vi "Periodic Tasks.vi"(8 "error in":errorcluster) -> ()   [LabVIEW 2014]
doc: "This VI runs in parallel to other tasks. It can contain as many user-defined periodic loops as you need. These can carry out PID or other sorts of timed response."
uses:
  <vilib>/Rock Robotics/WPI/Solenoid/WPI_SolenoidValue.ctl
  <vilib>/Rock Robotics/WPI/Relay/WPI_RelayValue.ctl
  <vilib>/Rock Robotics/WPI/DriverStation/WPI_DriverStationRobotMode2.ctl
  TORC Code/DriveSwitch.ctl
  Robot Global Data.vi
  TORC Code/GlobalVariable.vi
  <vilib>/Rock Robotics/WPI/Solenoid/WPI_SolenoidSetEnum.vi
  <vilib>/Rock Robotics/WPI/Solenoid/Deprecated/WPI_SolenoidGetBool.vi
  <vilib>/Rock Robotics/WPI/RobotDrive/WPI_RobotDriveGetSetRefNum.vi
  <vilib>/Rock Robotics/WPI/Joystick/WPI_JoystickGetSetRefNum.vi
  <vilib>/Rock Robotics/WPI/Compressor/WPI_CompressorGetSetRefNum.vi
  <vilib>/Rock Robotics/Network Tables/SD Write Numeric Array.vi
  <vilib>/Rock Robotics/Network Tables/SD Write Boolean Array.vi
  Moose Code/Auto_Conf.vi
panel:
  out "Right Distance":dbl
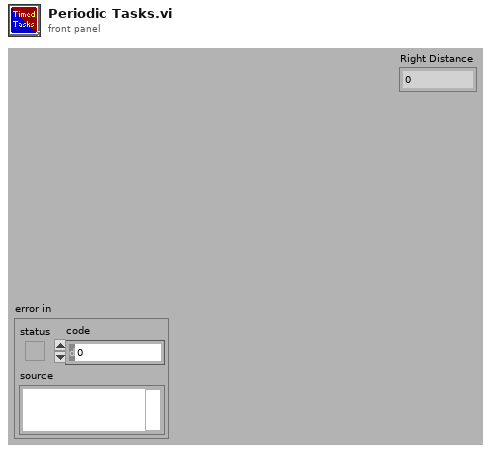
[diagram p1: front panel]
types:
  T1 = enum16{"Unready", "Ready", "Clear", "Fire", "Reload", "Arm In"}
  T2 = typedef "WPI_JoystickDevRef.ctl" = cluster{"Device":T3}
  T3 = typedef "WPI_JoystickDeviceEnum.ctl" = enum16{"USB 0", "USB 1", "USB 2", "USB 3", "USB 4", "USB 5"}
  T4 = typedef "WPI_SolenoidDevRef.ctl" = cluster{"DevStatus":errorcluster, "Pneumatics Control Module":u8, "Forward Solenoid Channel":T5, "Reverse Solenoid Channel":T5}
  T5 = typedef "WPI_SolenoidChannel.ctl" = enum8{"Solenoid 0", "Solenoid 1", "Solenoid 2", "Solenoid 3", "Solenoid 4", "Solenoid 5", "Solenoid 6", "Solenoid 7", "Invalid"}
  T6 = typedef "WPI_AnalogChannelDevRef.ctl" = cluster{"DevStatus":errorcluster, "Controller":T7, "Analog Channel":T8}
  T7 = typedef "FPGA_TypedefAnalogModule.ctl" = enum16{"Controller 1"}
  T8 = typedef "FPGA_AIChannel.ctl" = enum8{"AI 0", "AI 1", "AI 2", "AI 3", "AI MXP 0", "AI MXP 1", "AI MXP 2", "AI MXP 3", "Invalid"}
  T9 = typedef "WPI_DigitalInputDevRef.ctl" = cluster{"DevStatus":errorcluster, "DIO Channel":T10, "Controller":T11}
  T10 = typedef "FPGA_DIOChannel.ctl" = enum8{"DIO 0", "DIO 1", "DIO 2", "DIO 3", "DIO 4", "DIO 5", "DIO 6", "DIO 7", "DIO 8", "DIO 9", "DIO MXP 0", "DIO MXP 1", "DIO MXP 2", "DIO MXP 3", "DIO MXP 4", "DIO MXP 5", "DIO MXP 6", "DIO MXP 7", "DIO MXP 8", "DIO MXP 9", "DIO MXP 10", "DIO MXP 11", "DIO MXP 12", "DIO MXP 13", "DIO MXP 14", "DIO MXP 15", "Invalid"}
  T11 = typedef "FPGA_TypedefDigitalModule.ctl" = enum16{"Controller 1"}
  T12 = typedef "WPI_RobotDriveDevRef.ctl" = cluster{"DevStatus":errorcluster, "Motors[]":T13[], "Square Inputs":bool, "Max Output":dbl}
  T13 = typedef "WPI_MotorControlDeviceRef.ctl" = cluster{"DeviceStatus":errorcluster, "Type":T14, "PWM":cluster{"Controller":T11, "PWM Channel":T15, "DeadBand":T16}, "CAN":cluster{"Device Number":u8, "Control Mode":T17, "Semaphore":T18, "Max Vout":dbl, "TalonSRX Control Mode":T19}, "Invert":bool, "TransformRef":T20, "InvTransformRef":T20}
  T14 = typedef "WPI_MotorControlType.ctl" = enum16{"PWM", "CAN", "CANTalonSRX"}
  T15 = typedef "FPGA_DIOPWMChannel.ctl" = enum8{"PWM 0", "PWM 1", "PWM 2", "PWM 3", "PWM 4", "PWM 5", "PWM 6", "PWM 7", "PWM 8", "PWM 9", "PWM MXP 0", "PWM MXP 1", "PWM MXP 2", "PWM MXP 3", "PWM MXP 4", "PWM MXP 5", "PWM MXP 6", "PWM MXP 7", "PWM MXP 8", "PWM MXP 9", "Invalid"}
  T16 = typedef "WPI_PWMDeadband.ctl" = cluster{"Name":string, "maxPositivePwm":i32, "minPositivePwm":i32, "centerPwm":i32, "maxNegativePwm":i32, "minNegativePwm":i32, "angularRange":u16}
  T17 = typedef "WPI_CANJaguar_ControlMode.ctl" = enum8{"Percent VBus", "Current", "Speed", "Position", "Voltage"}
  T18 = typedef "Semaphore RefNum" = refnum<k1>
  T19 = typedef "WPI_CANTalonSRX_APIControlMode.ctl" = enum8{"Percent VBus", "Speed", "Position", "Slave", "Unchanged / Invalid"}
  T20 = typedef "WPI_PWMTransform_ConPane.ctl" = refnum<vi>
  T21 = typedef "WPI_GyroDevRef.ctl" = cluster{"DevStatus":errorcluster, "Analog Module":T7, "Analog Channel":T8, "Offset":dbl, "Gain (VoltsPerDegree/Second)":dbl}
  T22 = typedef "WPI_RelayDevRef.ctl" = cluster{"DevStatus":errorcluster, "Relay Channel":T23, "Controller":T11, "Relay Direction":T24}
  T23 = typedef "FPGA_DIORelayChannel.ctl" = enum8{"Relay 0", "Relay 1", "Relay 2", "Relay 3", "Invalid"}
  T24 = typedef "WPI_RelayDirection.ctl" = enum16{"Both directions", "Forward only", "Reverse only"}
  T25 = typedef "WPI_EncoderDevRef.ctl" = cluster{"DevStatus":errorcluster, "EncoderIndex":T26, "CounterIndex":T27, "DistancePerCount":dbl, "Decoding Type":T28}
  T26 = typedef "FPGA_EncoderIdx.ctl" = enum8{"Enc 0", "Enc 1", "Enc 2", "Enc 3", "Enc 4", "Enc 5", "Enc 6", "Enc 7", "Invalid"}
  T27 = typedef "FPGA_CounterCtrSystemIndex.ctl" = enum8{"Ctr 0", "Ctr 1", "Ctr 2", "Ctr 3", "Ctr 4", "Ctr 5", "Ctr 6", "Ctr 7", "Invalid"}
  T28 = typedef "WPI_EncoderType.ctl" = enum16{"1x", "2x", "4x"}
  T29 = typedef "WPI_CompressorDevRef.ctl" = cluster{"DevStatus":errorcluster, "Pneumatics Control Module":u8}
  T30 = typedef "WPI_DriverStationRobotMode2.ctl" = enum16{"Autonomous Disabled", "Autonomous Enabled", "Teleop Disabled", "Teleop Enabled", "Disconnected", "Finish", "Test Disabled", "Test Enabled", "Emergency Stopped"}
  T31 = typedef "WPI_RelayValue.ctl" = enum16{"Off", "On", "Forward", "Reverse"}
  T32 = typedef "WPI_SolenoidValue.ctl" = enum16{"Off", "On", "Forward", "Reverse"}
  T33 = cluster{"Buttons[0]":bool, "Buttons[1]":bool, "Buttons[2]":bool, "Buttons[3]":bool, "Buttons[4]":bool, "Buttons[5]":bool, "Buttons[6]":bool, "Buttons[7]":bool, "Buttons[8]":bool}
  T34 = typedef "DriveSwitch.ctl" = enum16{"High", "Low", "Auto"}
  T35 = typedef "Shift Enum.ctl" = enum16{"High", "Low"}
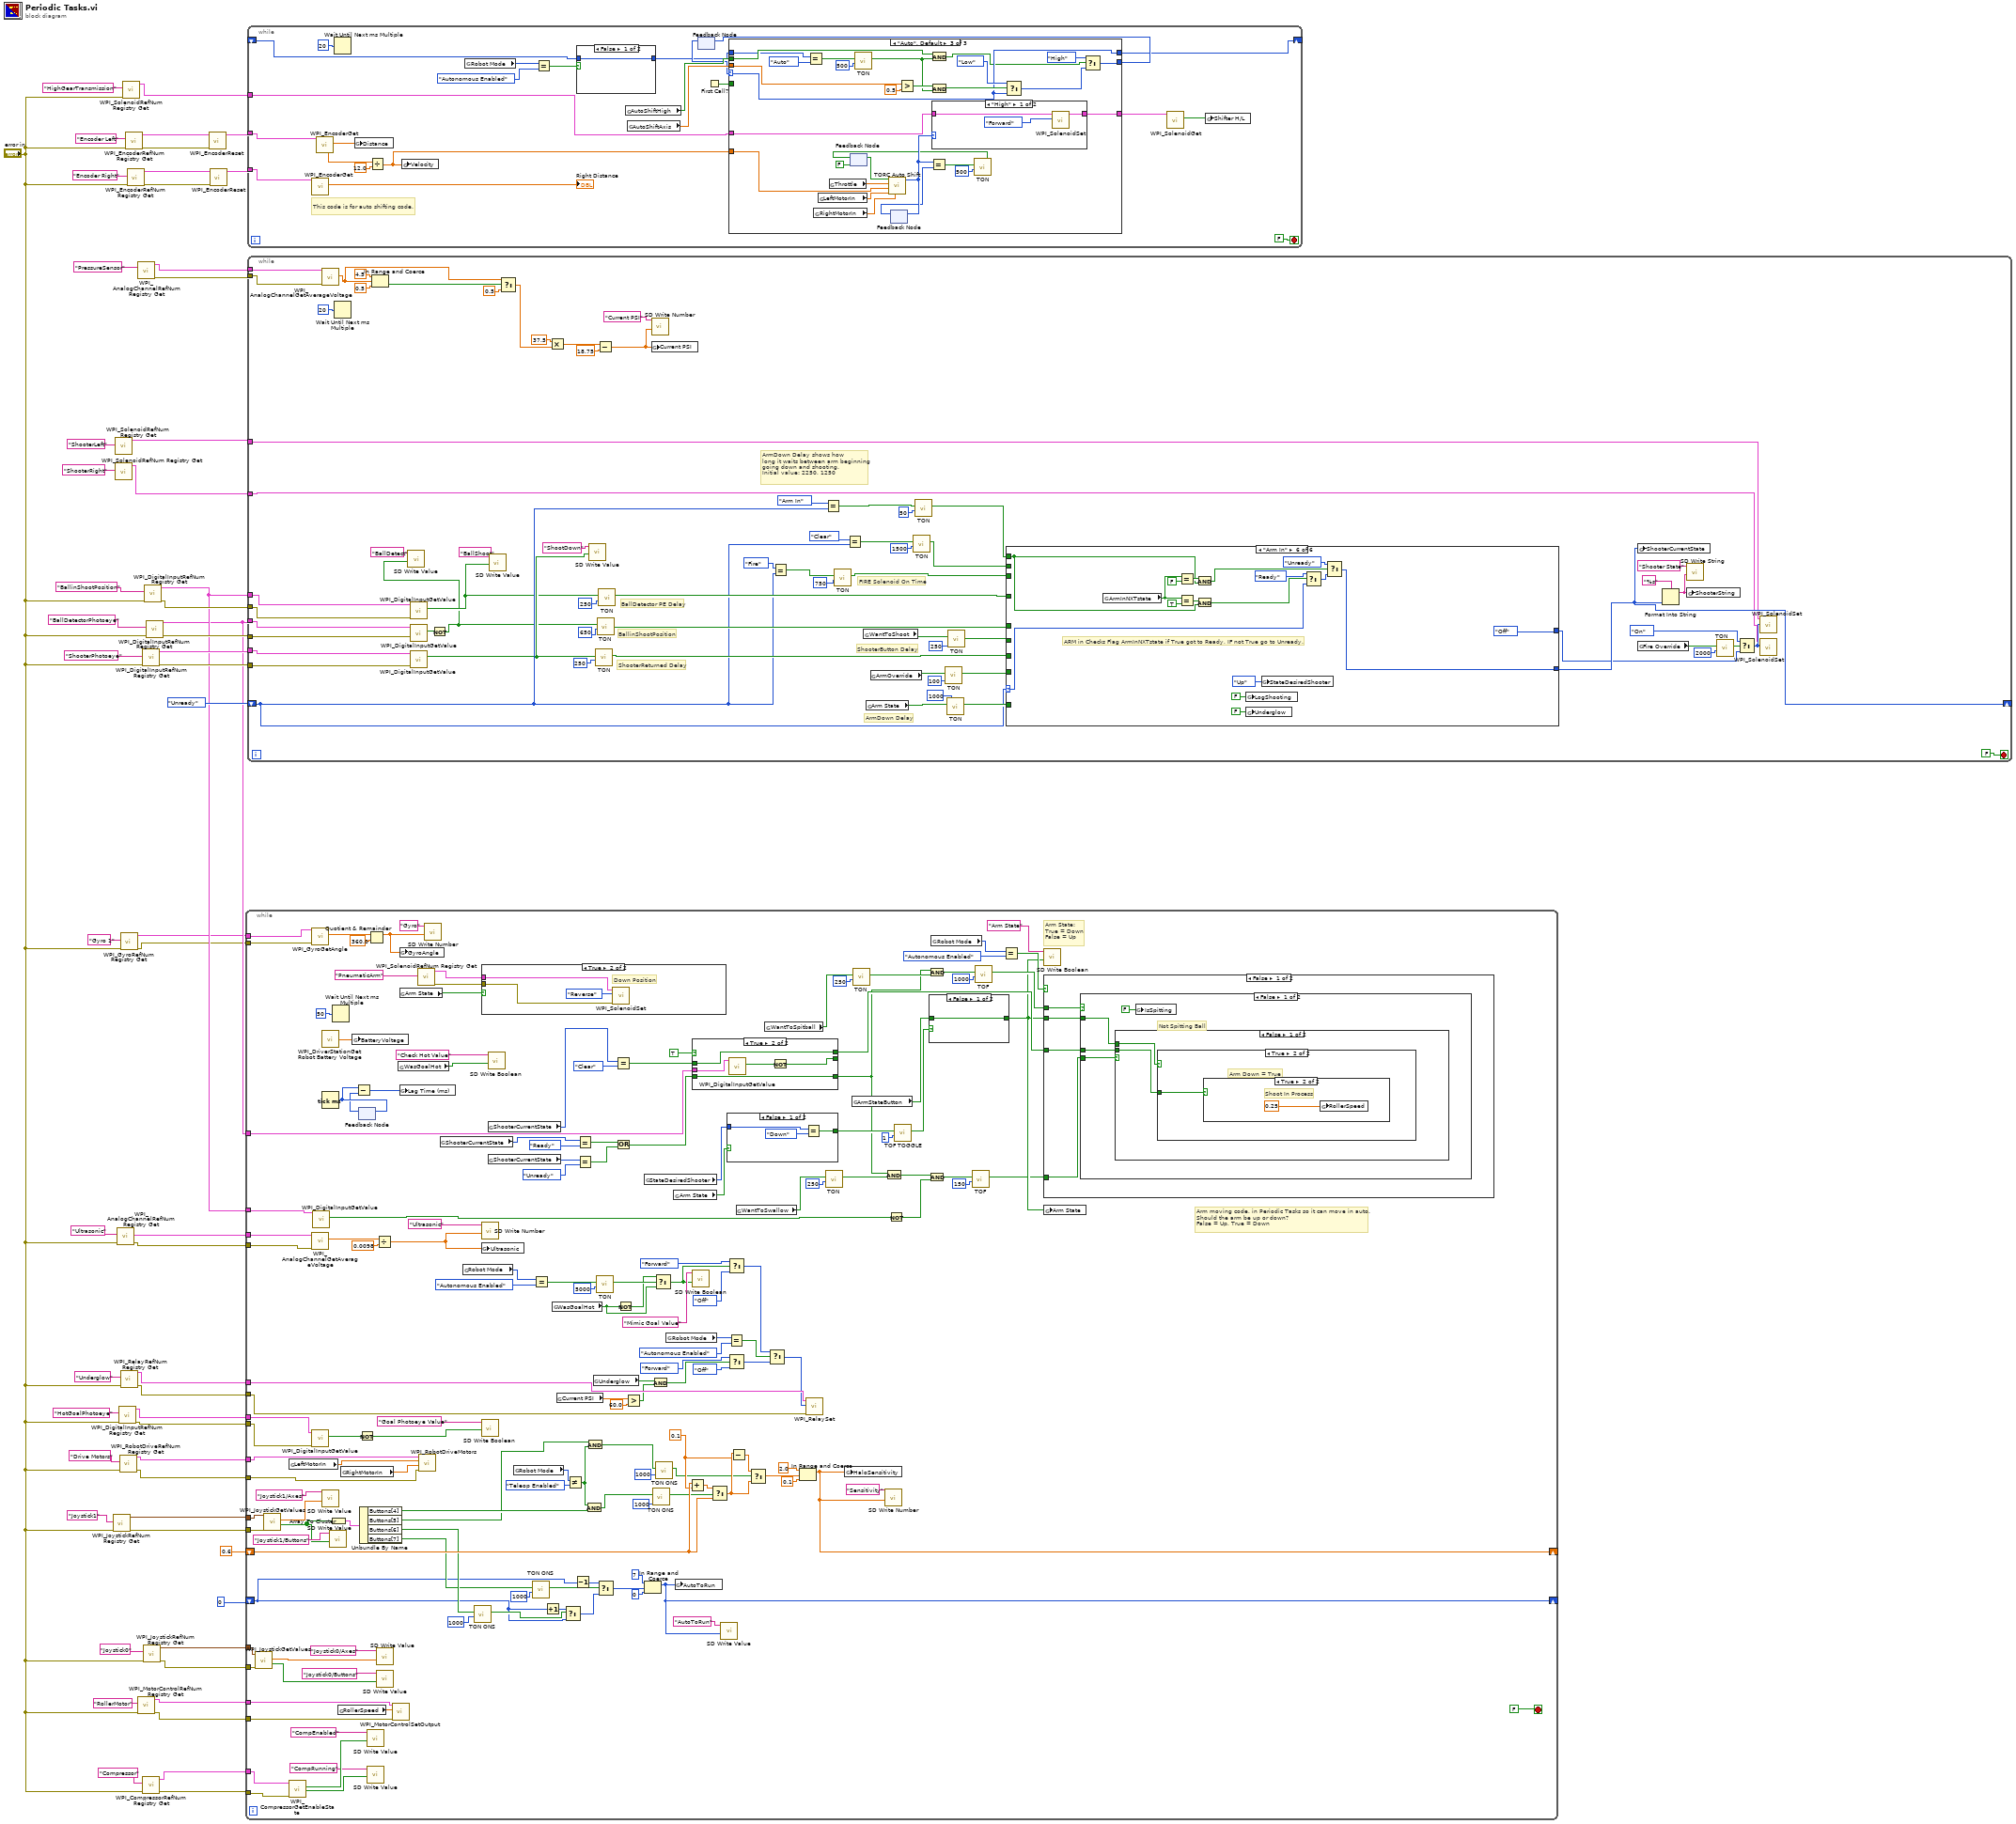
[diagram p0: block diagram]
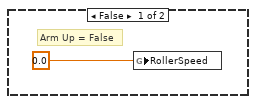
[diagram p2: hidden frame]
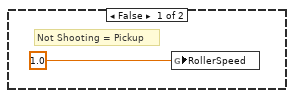
[diagram p3: hidden frame]
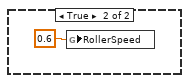
[diagram p4: hidden frame]
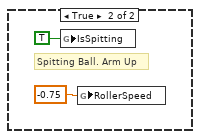
[diagram p5: hidden frame]
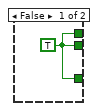
[diagram p7: hidden frame]
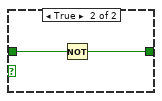
[diagram p8: hidden frame]
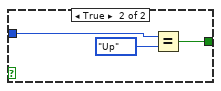
[diagram p9: hidden frame]
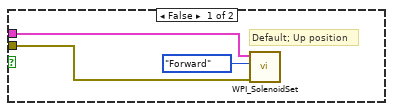
[diagram p10: hidden frame]
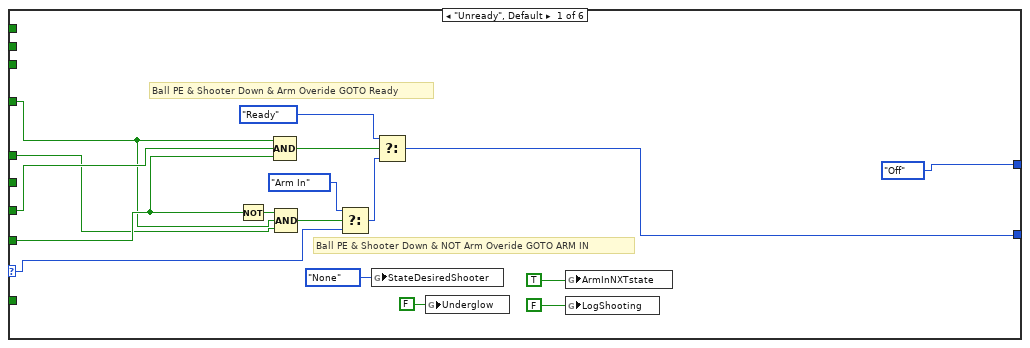
[diagram p11: hidden frame]
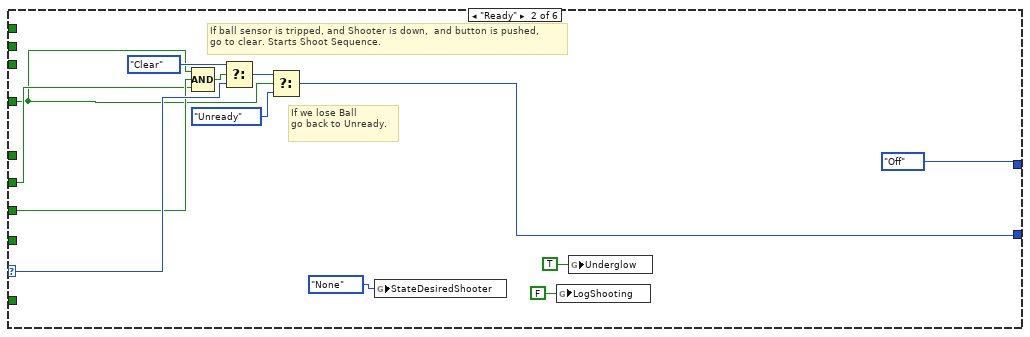
[diagram p12: hidden frame]
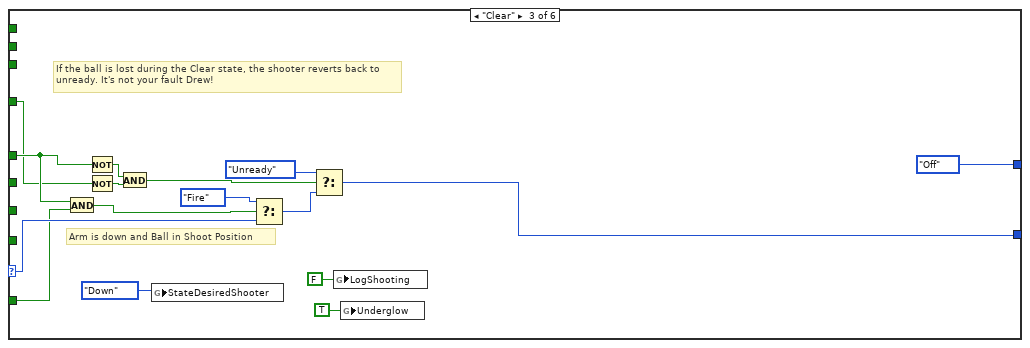
[diagram p13: hidden frame]
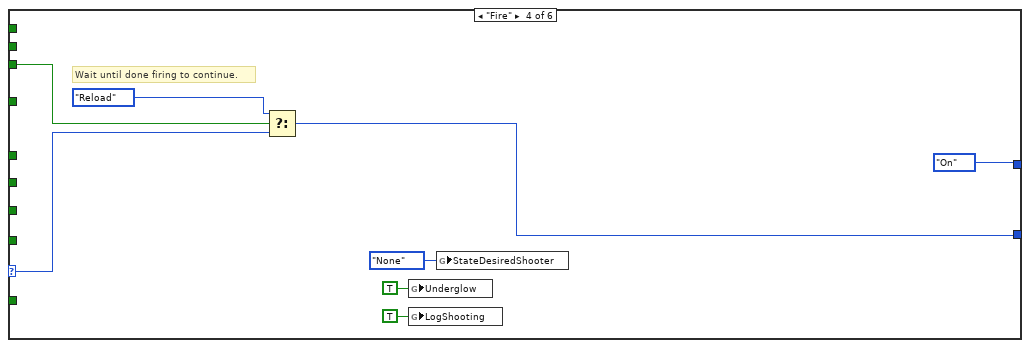
[diagram p14: hidden frame]
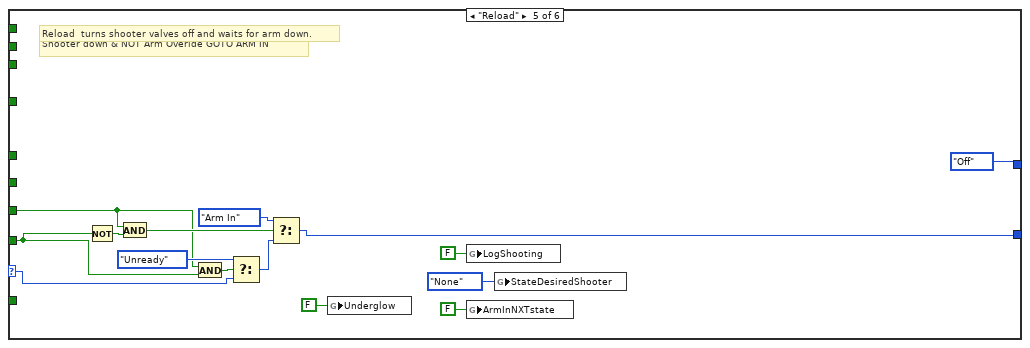
[diagram p15: hidden frame]
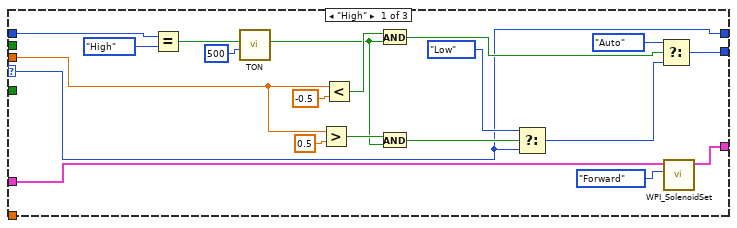
[diagram p16: hidden frame]
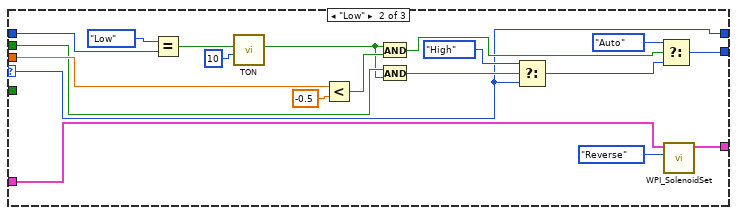
[diagram p17: hidden frame]
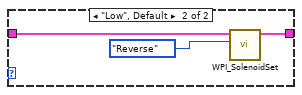
[diagram p18: hidden frame]
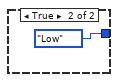
[diagram p19: hidden frame]
diagram:
  n1 = call <vilib>:"WPI_JoystickRefNum Registry Get.vi"("error in (no error)"="error in", "refnum name"="Joystick1") -> ("error out"=w1:errorcluster, "JoystickDevRef"=w9:T2)  [unwired: 8 in]
  n2 = call <vilib>:"WPI_SolenoidRefNum Registry Get.vi"("refnum name"="ShooterLeft") -> ("SolenoidDevRef"=w43:T4)  [unwired: 9 in, 1 out]
  n3 = call <vilib>:"WPI_SolenoidRefNum Registry Get.vi"("refnum name"="ShooterRight") -> ("SolenoidDevRef"=w44:T4)  [unwired: 9 in, 1 out]
  n4 = call <vilib>:"WPI_AnalogChannelRefNum Registry Get.vi"("error in (no error)"="error in", "refnum name"="Ultrasonic") -> ("error out"=w31:errorcluster, "AIDeviceRef"=w32:T6)  [unwired: 8 in]
  n5 = call <vilib>:"WPI_DigitalInputRefNum Registry Get.vi"("error in (no error)"="error in", "refnum name"="HotGoalPhotoeye") -> ("error out"=w17:errorcluster, "DigitalInputDevRef"=w18:T9)  [unwired: 8 in]
  n6 = call <vilib>:"WPI_RobotDriveRefNum Registry Get.vi"("error in (no error)"="error in", "refnum name"="Drive Motors") -> ("error out"=w25:errorcluster, "RobotDriveDevRef"=w26:T12)  [unwired: 8 out]
  n7 = call <vilib>:"WPI_GyroRefNum Registry Get.vi"("error in (no error)"="error in", "refnum name"="Gyro 1") -> ("error out"=w28:errorcluster, "GyroDevRef"=w29:T21)  [unwired: 8 in]
  n8 = call <vilib>:"WPI_RelayRefNum Registry Get.vi"("error in (no error)"="error in", "refnum name"="Underglow") -> ("error out"=w14:errorcluster, "RelayDevRef"=w15:T22)  [unwired: 8 in]
  n9 = call <vilib>:"WPI_SolenoidRefNum Registry Get.vi"("error in (no error)"="error in", "refnum name"="HighGearTransmission") -> ("SolenoidDevRef"=w50:T4)  [unwired: 8 in, 1 out]
  n10 = call <vilib>:"WPI_EncoderRefNum Registry Get.vi"("error in (no error)"="error in", "refnum name"="Encoder Left") -> ("error out"=w36:errorcluster, "EncoderDevRef"=w55:T25)  [unwired: 8 in]
  n11 = call <vilib>:"WPI_EncoderRefNum Registry Get.vi"("error in (no error)"="error in", "refnum name"="Encoder Right") -> ("error out"=w37:errorcluster, "EncoderDevRef"=w56:T25)  [unwired: 8 in]
  n12 = call <vilib>:"WPI_AnalogChannelRefNum Registry Get.vi"("refnum name"="PressureSensor") -> ("error out"=w6:errorcluster, "AIDeviceRef"=w7:T6)  [unwired: 9 in]
  n13 = call <vilib>:"WPI_MotorControlRefNum Registry Get.vi"("error in (no error)"="error in", "refnum name"="RollerMotor") -> ("error out"=w22:errorcluster, "MotorControlDevRef"=w23:T13)  [unwired: 8 in]
  n14 = call <vilib>:"WPI_DigitalInputRefNum Registry Get.vi"("error in (no error)"="error in", "refnum name"="ShooterPhotoeye") -> ("error out"=w39:errorcluster, "DigitalInputDevRef"=w42:T9)  [unwired: 8 in]
  n15 = call <vilib>:"WPI_CompressorRefNum Registry Get.vi"("error in (no error)"="error in", "refnum name"="Compressor") -> ("error out"=w11:errorcluster, "CompressorDevRef"=w12:T29)  [unwired: 8 in]
  n16 = call <vilib>:"WPI_JoystickRefNum Registry Get.vi"("error in (no error)"="error in", "refnum name"="Joystick0") -> ("error out"=w3:errorcluster, "JoystickDevRef"=w2:T2)  [unwired: 8 out]
  n17 = call <vilib>:"WPI_DigitalInputRefNum Registry Get.vi"("error in (no error)"="error in", "refnum name"="BallinShootPosition") -> ("error out"=w41:errorcluster, "DigitalInputDevRef"=w35:T9)  [unwired: 8 in]
  n18 = call <vilib>:"WPI_DigitalInputRefNum Registry Get.vi"("error in (no error)"="error in", "refnum name"="BallDetectorPhotoeye") -> ("error out"=w40:errorcluster, "DigitalInputDevRef"=w34:T9)  [unwired: 8 in]
  n19 = call <vilib>:"WPI_EncoderReset.vi"("error in (no error)"=w36, "EncoderDevRef"=w55) -> ("EncoderDevRef"=w52:T25)  [unwired: 8 in, 1 out]
  n20 = call <vilib>:"WPI_EncoderReset.vi"("error in (no error)"=w37, "EncoderDevRef"=w56) -> ("EncoderDevRef"=w51:T25)  [unwired: 8 in, 1 out]
  n21 = while {
    tunnel: w23 -> [w210]
    tunnel: w22 -> [w211]
    tunnel: w26 -> [w208]
    tunnel: w25 -> [w207]
    tunnel: w34 -> [w197]
    tunnel: w29 -> [w182]
    tunnel: w28 -> [w183]
    tunnel: w32 -> [w161]
    tunnel: w31 -> [w160]
    shift-right: [w78] -> _
    shift-left: u8 0 ("upper limit") -> [w80]
    shift-right: [w146] -> _
    shift-left: 0.6 ("upper limit") -> [w165]
    tunnel: w18 -> [w141]
    tunnel: w17 -> [w140]
    tunnel: w14 -> [w139]
    tunnel: w15 -> [w138]
    tunnel: w35 -> [w96]
    tunnel: w12 -> [w86]
    tunnel: w11 -> [w85]
    tunnel: w9 -> [w69]
    tunnel: w3 -> [w60]
    tunnel: w2 -> [w59]
    tunnel: w1 -> [w58]
    stop <- FALSE stop-if-true
    w162 = 0.1 ("y")
    # "Arm State:\nTrue = Down\nFalse = Up"
    # "Arm moving code, in Periodic Tasks so it can move in auto.\nShould the arm be up or down?\nFalse = Up, True = Down"
    n22 = call <vilib>:"WPI_JoystickGetValues.vi"("error in (no error)"=w60, "JoystickDevRef"=w59) -> ("Buttons"=w64:bool[], "Axes"=w63:dbl[])  [unwired: 5 in, 3 out]
    n23 = call <vilib>:"WPI_JoystickGetValues.vi"("error in (no error)"=w58, "JoystickDevRef"=w69) -> ("Buttons"=w65:bool[], "Axes"=w67:dbl[])  [unwired: 5 in, 3 out]
    n24 = global read "GlobalVariable.vi" "LeftMotorIn"() -> (w206:dbl)
    n25 = call <vilib>:"WPI_CompressorGetEnableState.vi"("error in (no error)"=w85, "CompressorDevRef"=w86) -> ("Compressor Running"=w83:bool, "Enabled"=w84:bool)  [unwired: 6 in, 2 out]
    n26 = call <vilib>:"WPI_GyroGetAngle.vi"("error in (no error)"=w183, "GyroDevRef"=w182) -> ("Angle"=w180:dbl)  [unwired: 6 in, 3 out]
    n27 = call <vilib>:"WPI_AnalogChannelGetAverageVoltage.vi"("error in (no error)"=w160, "AIDeviceRef"=w161) -> ("Voltage"=w159:dbl)  [unwired: 7 in, 2 out]
    n28 = call <vilib>:"WPI_DigitalInputGetValue.vi"("error in (no error)"=w140, "DigitalInputDevRef"=w141) -> ("Value"=w128:bool)  [unwired: 7 in, 2 out]
    n29 = call <vilib>:"WPI_DigitalInputGetValue.vi"("DigitalInputDevRef"=w96) -> ("Value"=w95:bool)  [unwired: 8 in, 2 out]
    n30 = call <vilib>:"WPI_DriverStationGet Robot Battery Voltage.vi"() -> ("robot battery voltage"=w151:dbl)  [unwired: 14 in, 1 out]
    n31 = Tick Count (ms)() -> (millisecond timer value=w150:u32)
    n32 = call-poly <vilib>:"SD Write Value.vi"("Numeric Array"=w67, "Name"="Joystick1/Axes") -> ()  [unwired: 8 in, 2 out]
    n33 = call-poly <vilib>:"SD Write Value.vi"("Boolean Array"=w65, "Name"="Joystick1/Buttons") -> ()  [unwired: 8 in, 2 out]
    n34 = Array To Cluster(array=w65) -> (cluster=w93:T33)
    n35 = Wait Until Next ms Multiple(millisecond multiple=u32 50) -> ()  [unwired: 1 out]
    n36 = global read "GlobalVariable.vi" "RollerSpeed"() -> (w193:dbl)
    n37 = global read "GlobalVariable.vi" "RightMotorIn"() -> (w205:dbl)
    n38 = global write "GlobalVariable.vi" "BatteryVoltage"(w151) -> ()
    n39 = feedback-in #1(w150) -> ()
    n40 = feedback #1() -> (w149:u32)  [unwired: 1 in]
    n41 = Subtract(x=w150, y=w149) -> (x-y=w148:u32)
    n42 = Not(x=w128) -> (.not. x?=w135:bool)
    n43 = Unbundle By Name(w93) -> ("Buttons[4]"=w74:bool, "Buttons[5]"=w70:bool, "Buttons[6]"=w155:bool, "Buttons[7]"=w152:bool)
    n44 = call-poly <vilib>:"SD Write Value.vi"("Boolean"=w84, "Name"="CompEnabled") -> ()  [unwired: 8 in, 2 out]
    n45 = call-poly <vilib>:"SD Write Value.vi"("Boolean"=w83, "Name"="CompRunning") -> ()  [unwired: 8 in, 2 out]
    n46 = Quotient & Remainder(x=w180, y=360.0) -> (x-y*floor(x/y)=w88:dbl)  [unwired: 1 out]
    n47 = Divide(x=w159, y=0.0098) -> (x/y=w157:dbl)
    n48 = call-poly <vilib>:"SD Write Value.vi"("Numeric Array"=w63, "Name"="Joystick0/Axes") -> ()  [unwired: 8 in, 2 out]
    n49 = call-poly <vilib>:"SD Write Value.vi"("Boolean Array"=w64, "Name"="Joystick0/Buttons") -> ()  [unwired: 8 in, 2 out]
    n50 = call <vilib>:"WPI_MotorControlSetOutput.vi"("error in (no error)"=w211, "Output"=w193, "MotorControlDevRef"=w210) -> ()  [unwired: 6 in, 3 out]
    n51 = global read "GlobalVariable.vi" "WasGoalHot"() -> (w136:bool)
    n52 = global write "GlobalVariable.vi" "GyroAngle"(w88) -> ()
    n53 = global read "GlobalVariable.vi" "Arm State"() -> (w194:bool)
    n54 = global write "GlobalVariable.vi" "Lag Time (ms)"(w148) -> ()
    n55 = call <vilib>:"WPI_SolenoidRefNum Registry Get.vi"("refnum name"="PneumaticArm") -> ("error out"=w214:errorcluster, "SolenoidDevRef"=w212:T4)  [unwired: 9 in]
    n56 = call <vilib>:"WPI_RobotDriveMotors.vi"("error in (no error)"=w207, "RightSpeed"=w205, "LeftSpeed"=w206, "RobotDriveDevRef"=w208) -> ()  [unwired: 8 out]
    n57 = call <vilib>:"SD Write Number.vi"("Numeric"=w88, "Name"="Gyro") -> ()  [unwired: 8 in, 2 out]
    n58 = global read "GlobalVariable.vi" "ShooterCurrentState"() -> (w192:T1)
    n59 = global read "Robot Global Data.vi" "Robot Mode"() -> (w118:T30)
    n60 = call "TON ONS.vi"("Delay (ms)"=u32 1000 ("Delay ms"), "Input"=w155) -> ("Output 2"=w154:bool)  [unwired: 9 in]
    n61 = case shown="True" w194 {
      tunnel: w212 -> [w249 w253]
      tunnel: w214 -> [w248 w251]
      frame False {
        # "Default; Up position"
        n62 = call-poly <vilib>:"WPI_SolenoidSet.vi"("error in (no error)"=w248, "Value"=WPI_SolenoidValue."Forward", "SolenoidDevRef"=w249) -> ()  [unwired: 7 in, 2 out]
      }
      frame True {
        # "Down Position"
        n63 = call-poly <vilib>:"WPI_SolenoidSet.vi"("error in (no error)"=w251, "Value"=WPI_SolenoidValue."Reverse", "SolenoidDevRef"=w253) -> ()  [unwired: 7 in, 2 out]
      }
    }
    n64 = call <vilib>:"SD Write Number.vi"("Numeric"=w157, "Name"="Ultrasonic") -> ()  [unwired: 8 in, 2 out]
    n65 = global write "GlobalVariable.vi" "Ultrasonic"(w157) -> ()
    n66 = call <vilib>:"SD Write Boolean.vi"("Boolean"=w135, "Name"="Goal Photoeye Value") -> ()  [unwired: 8 in, 2 out]
    n67 = call <vilib>:"SD Write Boolean.vi"("Boolean"=w136, "Name"="Check Hot Value") -> ()  [unwired: 8 in, 2 out]
    n68 = global read "GlobalVariable.vi" "ShooterCurrentState"() -> (w187:T1)
    n69 = global read "GlobalVariable.vi" "ShooterCurrentState"() -> (w108:T1)
    n70 = global read "Robot Global Data.vi" "Robot Mode"() -> (w92:T30)
    n71 = call "TON ONS.vi"("Delay (ms)"=u32 1000 ("Delay ms"), "Input"=w152) -> ("Output 2"=w153:bool)  [unwired: 9 in]
    n72 = Equal?(x=w118, y=WPI_DriverStationRobotMode2."Autonomous Enabled") -> (x = y?=w116:bool)
    n73 = Increment(x=w80) -> (x+1=w176:u8)
    n74 = global read "GlobalVariable.vi" "WasGoalHot"() -> (w119:bool)
    n75 = global read "GlobalVariable.vi" "Current PSI"() -> (w123:dbl)
    n76 = Select(t=w176, s=w154, f=w80) -> (s? t:f=w175:u8)
    n77 = Not Equal?(x=w92, y=WPI_DriverStationRobotMode2."Teleop Enabled") -> (x != y?=w71:bool)
    n78 = Decrement(x=w80) -> (x-1=w174:u8)
    n79 = Equal?(x=w192, y=T1."Ready") -> (x = y?=w110:bool)
    n80 = Equal?(x=w108, y=T1."Unready") -> (x = y?=w107:bool)
    n81 = And(x=w71, y=w74) -> (x .and. y?=w73:bool)
    n82 = And(x=w70, y=w71) -> (x .and. y?=w90:bool)
    n83 = global read "GlobalVariable.vi" "Underglow"() -> (w129:bool)
    n84 = call "TON.vi"("Delay (ms)"=u32 5000 ("Delay ms"), "Input"=w116) -> ("Output"=w122:bool)  [unwired: 9 in]
    n85 = Select(t=w174, s=w153, f=w175) -> (s? t:f=w173:u8)
    n86 = Equal?(x=w187, y=T1."Clear") -> (x = y?=w185:bool)
    n87 = Or(x=w110, y=w107) -> (x .or. y?=w106:bool)
    n88 = Not(x=w119) -> (.not. x?=w120:bool)
    n89 = Greater?(x=w123, y=60.0) -> (0:w125:bool)
    n90 = global read "GlobalVariable.vi" "StateDesiredShooter"() -> (w203:enum16{"None", "Down", "Up"})
    n91 = In Range and Coerce(upper limit=u8 7, x=w173, lower limit=u8 0) -> (coerced(x)=w78:u8)  [unwired: 1 out]
    n92 = And(x=w129, y=w125) -> (x .and. y?=w126:bool)
    n93 = call "TON ONS.vi"("Delay (ms)"=u32 1000 ("Delay ms"), "Input"=w73) -> ("Output 2"=w72:bool)  [unwired: 9 in]
    n94 = Select(t=w120, s=w122, f=w119) -> (s? t:f=w114:bool)
    n95 = call "TON ONS.vi"("Delay (ms)"=u32 1000 ("Delay ms"), "Input"=w90) -> ("Output 2"=w156:bool)  [unwired: 9 in]
    n96 = global read "Robot Global Data.vi" "Robot Mode"() -> (w112:T30)
    n97 = global read "GlobalVariable.vi" "Arm State"() -> (w204:bool)
    n98 = global write "Auto_Conf.vi" "AutoToRun"(w78) -> ()
    n99 = Add(x=w165, y=w162) -> (x+y=w169:dbl)
    n100 = case shown="True" TRUE {
      tunnel: w197 -> [_ w238]
      tunnel: [w233 w234] -> _
      tunnel: [w233 w236] -> w104
      tunnel: w106 -> [_ w236]
      tunnel: w185 -> [_ w235]
      tunnel: [w233 w235] -> w184
      frame False {
        w233 = TRUE ("Value")
      }
      frame True {
        n101 = call <vilib>:"WPI_DigitalInputGetValue.vi"("DigitalInputDevRef"=w238) -> ("Value"=w237:bool)  [unwired: 8 in, 2 out]
        n102 = Not(x=w237) -> (.not. x?=w234:bool)
      }
    }
    n103 = call <vilib>:"SD Write Boolean.vi"("Boolean"=w114, "Name"="Mimic Goal Value") -> ()  [unwired: 8 in, 2 out]
    n104 = Select(t=w169, s=w72, f=w165) -> (s? t:f=w166:dbl)
    n105 = call-poly <vilib>:"SD Write Value.vi"("Numeric"=w78, "Name"="AutoToRun") -> ()  [unwired: 8 in, 2 out]
    n106 = case shown="False" w204 {
      tunnel: w203 -> [w243 w247]
      tunnel: [w242 w245] -> w196
      frame False {
        n107 = Equal?(x=w243, y=enum16{"None", "Down", "Up"}."Down") -> (x = y?=w242:bool)
      }
      frame True {
        n108 = Equal?(x=w247, y=enum16{"None", "Down", "Up"}."Up") -> (x = y?=w245:bool)
      }
    }
    n109 = Select(t=WPI_RelayValue."Forward" ("RelayValue"), s=w114, f=WPI_RelayValue."Off" ("RelayValue")) -> (s? t:f=w134:T31)
    n110 = Equal?(x=w112, y=WPI_DriverStationRobotMode2."Autonomous Enabled") -> (x = y?=w111:bool)
    n111 = Select(t=WPI_RelayValue."Forward" ("RelayValue"), s=w126, f=WPI_RelayValue."Off" ("RelayValue")) -> (s? t:f=w127:T31)
    n112 = Subtract(x=w166, y=w162) -> (x-y=w168:dbl)
    n113 = global read "GlobalVariable.vi" "WantToSwallow"() -> (w102:bool)
    n114 = Select(t=w168, s=w156, f=w166) -> (s? t:f=w167:dbl)
    n115 = global read "GlobalVariable.vi" "WantToSpitball"() -> (w199:bool)
    n116 = Select(t=w134, s=w111, f=w127) -> (s? t:f=w137:T31)
    n117 = In Range and Coerce(upper limit=2.0, x=w167, lower limit=0.1) -> (coerced(x)=w146:dbl)  [unwired: 1 out]
    n118 = call <vilib>:"WPI_RelaySet.vi"("error in (no error)"=w139, "RelayValue"=w137, "RelayDevRef"=w138) -> ()  [unwired: 7 in, 2 out]
    n119 = call "TON.vi"("Delay (ms)"=u32 250 ("Delay ms"), "Input"=w102) -> ("Output"=w101:bool)  [unwired: 9 in]
    n120 = global write "GlobalVariable.vi" "HaloSensitivity"(w146) -> ()
    n121 = global read "GlobalVariable.vi" "ArmStateButton"() -> (w200:bool)
    n122 = call "TON.vi"("Delay (ms)"=u32 250 ("Delay ms"), "Input"=w199) -> ("Output"=w195:bool)  [unwired: 9 in]
    n123 = call <vilib>:"SD Write Number.vi"("Numeric"=w146, "Name"="Sensitivity") -> ()  [unwired: 8 in, 2 out]
    n124 = And(x=w104, y=w101) -> (x .and. y?=w100:bool)
    n125 = Not(x=w95) -> (.not. x?=w97:bool)
    n126 = call "TOF TOGGLE.vi"("Delay (ms)"=u32 1 ("Delay ms"), "Input"=w196) -> ("Output"=w202:bool)  [unwired: 9 in]
    n127 = And(x=w104, y=w195) -> (x .and. y?=w189:bool)
    n128 = And(x=w100, y=w97) -> (x .and. y?=w99:bool)
    n129 = case shown="False" w202 {
      tunnel: w200 -> [w239 w241]
      tunnel: [w239 w240] -> w144
      frame False {
      }
      frame True {
        n130 = Not(x=w241) -> (.not. x?=w240:bool)
      }
    }
    n131 = global read "Robot Global Data.vi" "Robot Mode"() -> (w179:T30)
    n132 = call "TOF.vi"("Delay (ms)"=u32 150 ("Delay ms"), "Input"=w99) -> ("Output"=w98:bool)  [unwired: 9 in]
    n133 = call "TOF.vi"("Delay (ms)"=u32 1000 ("Delay ms"), "Input"=w189) -> ("Output"=w188:bool)  [unwired: 9 in]
    n134 = Equal?(x=w179, y=WPI_DriverStationRobotMode2."Autonomous Enabled") -> (x = y?=w177:bool)
    n135 = call <vilib>:"SD Write Boolean.vi"("Boolean"=w144, "Name"="Arm State") -> ()  [unwired: 8 in, 2 out]
    n136 = case shown="False" w177 {
      tunnel: w188 -> [w219 _]
      tunnel: w144 -> [w218 _]
      tunnel: w184 -> [w217 _]
      tunnel: w98 -> [w216 _]
      frame False {
        n137 = case shown="False" w219 {
          tunnel: w218 -> [w223 _]
          tunnel: w217 -> [w221 _]
          tunnel: w216 -> [w220 _]
          frame False {
            # "Not Spitting Ball"
            n138 = case shown="False" w220 {
              tunnel: w223 -> [w225 _]
              tunnel: w221 -> [w224 _]
              frame False {
                n139 = case shown="True" w225 {
                  tunnel: w224 -> [_ w227]
                  frame False {
                    # "Arm Up = False"
                    n140 = global write "GlobalVariable.vi" "RollerSpeed"(0.0 ("RollerSpeed")) -> ()
                  }
                  frame True {
                    # "Arm Down = True"
                    n141 = case shown="True" w227 {
                      frame False {
                        # "Not Shooting = Pickup"
                        n142 = global write "GlobalVariable.vi" "RollerSpeed"(1.0 ("RollerSpeed")) -> ()
                      }
                      frame True {
                        # "Shoot In Process"
                        n143 = global write "GlobalVariable.vi" "RollerSpeed"(0.25 ("RollerSpeed")) -> ()
                      }
                    }
                  }
                }
              }
              frame True {
                n144 = global write "GlobalVariable.vi" "RollerSpeed"(0.6 ("RollerSpeed")) -> ()
              }
            }
            n145 = global write "GlobalVariable.vi" "IsSpitting"(FALSE ("IsSpitting")) -> ()
          }
          frame True {
            # "Spitting Ball. Arm Up"
            n146 = global write "GlobalVariable.vi" "IsSpitting"(TRUE ("IsSpitting")) -> ()
            n147 = global write "GlobalVariable.vi" "RollerSpeed"(-0.75 ("RollerSpeed")) -> ()
          }
        }
      }
      frame True {
      }
    }
    n148 = global write "GlobalVariable.vi" "Arm State"(w144) -> ()
  }
  n149 = while {
    shift-right: [w254] -> _
    shift-left: _ -> [w271]
    tunnel: w52 -> [w266]
    tunnel: w51 -> [w265]
    tunnel: w50 -> [w259]
    stop <- FALSE stop-if-true
    # "This code is for auto shifting code."
    n150 = call <vilib>:"WPI_EncoderGet.vi"("EncoderDevRef"=w265) -> ("Distance"=→"Right Distance":dbl)  [unwired: 5 in, 5 out]
    n151 = call <vilib>:"WPI_EncoderGet.vi"("EncoderDevRef"=w266) -> ("Distance"=w270:dbl, "Rate"=w267:dbl)  [unwired: 5 in, 4 out]
    n152 = Wait Until Next ms Multiple(millisecond multiple=u32 20 ("milliseconds to wait")) -> ()  [unwired: 1 out]
    n153 = global write "GlobalVariable.vi" "Distance"(w270) -> ()
    n154 = Divide(x=w267, y=12.0) -> (x/y=w258:dbl)
    n155 = global write "GlobalVariable.vi" "Velocity"(w258) -> ()
    n156 = global read "Robot Global Data.vi" "Robot Mode"() -> (w273:T30)
    n157 = Equal?(x=w273, y=WPI_DriverStationRobotMode2."Autonomous Enabled") -> (x = y?=w272:bool)
    n158 = case shown="False" w272 {
      tunnel: w271 -> [w351 _]
      tunnel: [w351 DriveSwitch."Low"] -> w255
      frame False {
      }
      frame True {
      }
    }
    n159 = global read "GlobalVariable.vi" "AutoShiftHigh"() -> (w260:bool)
    n160 = global read "GlobalVariable.vi" "AutoShiftAxis"() -> (w261:dbl)
    n161 = feedback #2() -> (w257:T34)  [unwired: 1 in]
    n162 = First Call?() -> (First Call?: T/F=w262:bool)
    n163 = case shown="\"Auto\", Default" w257 {
      selector: w257 -> [w279 w299 w328]
      tunnel: [w292 w311 w341] -> w256
      tunnel: w260 -> [_ w302 w331]
      tunnel: w259 -> [w290 w310 w337]
      tunnel: w261 -> [w288 w308 w336]
      tunnel: [w279 w299 w328] -> w254
      tunnel: w255 -> [w278 w298 w327]
      tunnel: w258 -> [_ _ w325]
      tunnel: [w277 w297 w326] -> w264
      tunnel: w262 -> [_ _ _]
      frame "High" {
        n164 = Equal?(x=w278, y=DriveSwitch."High") -> (x = y?=w286:bool)
        n165 = call "TON.vi"("Delay (ms)"=u32 500 ("Delay ms"), "Input"=w286) -> ("Output"=w280:bool)  [unwired: 9 in]
        n166 = Greater?(x=w288, y=0.5) -> (0:w282:bool)
        n167 = Less?(x=w288, y=-0.5) -> (x < y?=w281:bool)
        n168 = And(x=w281, y=w280) -> (x .and. y?=w284:bool)
        n169 = And(x=w282, y=w280) -> (x .and. y?=w283:bool)
        n170 = Select(t=DriveSwitch."Low", s=w283, f=w279) -> (s? t:f=w294:T34)
        n171 = Select(t=DriveSwitch."Auto", s=w284, f=w294) -> (s? t:f=w292:T34)
        n172 = call-poly <vilib>:"WPI_SolenoidSet.vi"("Value"=WPI_SolenoidValue."Forward", "SolenoidDevRef"=w290) -> ("SolenoidDevRef"=w277:T4)  [unwired: 8 in, 1 out]
      }
      frame "Low" {
        n173 = Equal?(x=DriveSwitch."Low", y=w298) -> (x = y?=w306:bool)
        n174 = call "TON.vi"("Delay (ms)"=u32 10 ("Delay ms"), "Input"=w306) -> ("Output"=w300:bool)  [unwired: 9 in]
        n175 = Less?(x=w308, y=-0.5) -> (x < y?=w301:bool)
        n176 = And(x=w300, y=w301) -> (x .and. y?=w304:bool)
        n177 = And(x=w302, y=w300) -> (x .and. y?=w303:bool)
        n178 = Select(t=DriveSwitch."High", s=w303, f=w299) -> (s? t:f=w313:T34)
        n179 = Select(t=DriveSwitch."Auto", s=w304, f=w313) -> (s? t:f=w311:T34)
        n180 = call-poly <vilib>:"WPI_SolenoidSet.vi"("Value"=WPI_SolenoidValue."Reverse", "SolenoidDevRef"=w310) -> ("SolenoidDevRef"=w297:T4)  [unwired: 8 in, 1 out]
      }
      frame "Auto", Default {
        n181 = Equal?(x=w327, y=DriveSwitch."Auto") -> (x = y?=w333:bool)
        n182 = global read "GlobalVariable.vi" "RightMotorIn"() -> (w339:dbl)
        n183 = global read "GlobalVariable.vi" "LeftMotorIn"() -> (w338:dbl)
        n184 = global read "GlobalVariable.vi" "Throttle"() -> (w324:dbl)
        n185 = feedback #3(FALSE ("DOUT-TON")) -> (w318:bool)
        n186 = call "TON.vi"("Delay (ms)"=u32 500 ("Delay ms"), "Input"=w333) -> ("Output"=w329:bool)  [unwired: 9 in]
        n187 = call "TORC Auto Shift.vi"("RightMotorInput"=w339, "Left Motor Input"=w338, "Velocity"=w325, "Throttle"=w324, "Time Met"=w318) -> ("Shift Indicator"=w323:T35)  [unwired: 6 in]
        n188 = feedback-in #4(w323) -> ()
        n189 = feedback #4() -> (w322:T35)  [unwired: 1 in]
        n190 = Greater?(x=w336, y=0.5) -> (0:w332:bool)
        n191 = Equal?(x=w323, y=w322) -> (x = y?=w321:bool)
        n192 = And(x=w331, y=w329) -> (x .and. y?=w316:bool)
        n193 = And(x=w332, y=w329) -> (x .and. y?=w335:bool)
        n194 = case shown="\"High\"" w323 {
          tunnel: w337 -> [w346 w350]
          tunnel: [w345 w348] -> w326
          frame "High" {
            n195 = call-poly <vilib>:"WPI_SolenoidSet.vi"("Value"=WPI_SolenoidValue."Forward", "SolenoidDevRef"=w346) -> ("SolenoidDevRef"=w345:T4)  [unwired: 8 in, 1 out]
          }
          frame "Low", Default {
            n196 = call-poly <vilib>:"WPI_SolenoidSet.vi"("Value"=WPI_SolenoidValue."Reverse", "SolenoidDevRef"=w350) -> ("SolenoidDevRef"=w348:T4)  [unwired: 8 in, 1 out]
          }
        }
        n197 = call "TON.vi"("Delay (ms)"=u32 500 ("Delay ms"), "Input"=w321) -> ("Output"=w319:bool)  [unwired: 9 in]
        n198 = feedback-in #3(w319) -> ()
        n199 = Select(t=DriveSwitch."Low", s=w335, f=w328) -> (s? t:f=w342:T34)
        n200 = Select(t=DriveSwitch."High", s=w316, f=w342) -> (s? t:f=w341:T34)
      }
    }
    n201 = feedback-in #2(w256) -> ()
    n202 = call-poly <vilib>:"WPI_SolenoidGet.vi"("SolenoidDevRef"=w264) -> ("Value"=w263:bool)  [unwired: 8 in, 2 out]
    n203 = global write "GlobalVariable.vi" "Shifter H/L"(w263) -> ()
  }
  n204 = while {
    shift-right: [w396] -> _
    shift-left: T1."Unready" ("t") -> [w360]
    tunnel: w34 -> [w364]
    tunnel: w40 -> [w363]
    tunnel: w42 -> [w362]
    tunnel: w39 -> [w361]
    tunnel: w43 -> [w377]
    tunnel: w44 -> [w370]
    tunnel: w35 -> [w366]
    tunnel: w41 -> [w365]
    tunnel: w7 -> [w359]
    tunnel: w6 -> [w358]
    stop <- FALSE stop-if-true
    # "ArmDown Delay shows how\nlong it waits between arm beginning\ngoing down and shooting.\nInitial value: 2250, 1250"
    # "BallinShootPosition"
    # "FIRE Solenoid On Time"
    # "ArmDown Delay"
    # "ShooterButton Delay"
    # "ShooterReturned Delay"
    # "BallDetector PE Delay"
    n205 = call <vilib>:"WPI_AnalogChannelGetAverageVoltage.vi"("error in (no error)"=w358, "AIDeviceRef"=w359) -> ("Voltage"=w357:dbl)  [unwired: 7 in, 2 out]
    n206 = Wait Until Next ms Multiple(millisecond multiple=u32 20) -> ()  [unwired: 1 out]
    n207 = In Range and Coerce(upper limit=4.5, x=w357, lower limit=0.5) -> (In Range?=w384:bool)  [unwired: 1 out]
    n208 = call <vilib>:"WPI_DigitalInputGetValue.vi"("error in (no error)"=w365, "DigitalInputDevRef"=w366) -> ("Value"=w355:bool)  [unwired: 7 in, 2 out]
    n209 = call <vilib>:"WPI_DigitalInputGetValue.vi"("error in (no error)"=w361, "DigitalInputDevRef"=w362) -> ("Value"=w356:bool)  [unwired: 7 in, 2 out]
    n210 = call <vilib>:"WPI_DigitalInputGetValue.vi"("error in (no error)"=w363, "DigitalInputDevRef"=w364) -> ("Value"=w354:bool)  [unwired: 7 in, 2 out]
    n211 = Not(x=w354) -> (.not. x?=w353:bool)
    n212 = call-poly <vilib>:"SD Write Value.vi"("Boolean"=w353, "Name"="BallDetect") -> ()  [unwired: 8 in, 2 out]
    n213 = call-poly <vilib>:"SD Write Value.vi"("Boolean"=w355, "Name"="BallShoot") -> ()  [unwired: 8 in, 2 out]
    n214 = Select(t=w357, s=w384, f=0.5) -> (s? t:f=w383:dbl)
    n215 = Multiply(x=37.5, y=w383) -> (x*y=w391:dbl)
    n216 = call-poly <vilib>:"SD Write Value.vi"("Boolean"=w356, "Name"="ShootDown") -> ()  [unwired: 8 in, 2 out]
    n217 = call "TON.vi"("Delay (ms)"=u32 250 ("Delay ms"), "Input"=w356) -> ("Output"=w408:bool)  [unwired: 9 in]
    n218 = Subtract(x=w391, y=18.75) -> (x-y=w388:dbl)
    n219 = call "TON.vi"("Delay (ms)"=u32 650 ("Delay ms"), "Input"=w353) -> ("Output"=w400:bool)  [unwired: 9 in]
    n220 = call "TON.vi"("Delay (ms)"=u32 250 ("Delay ms"), "Input"=w355) -> ("Output"=w403:bool)  [unwired: 9 in]
    n221 = call <vilib>:"SD Write Number.vi"("Numeric"=w388, "Name"="Current PSI") -> ()  [unwired: 8 in, 2 out]
    n222 = global write "GlobalVariable.vi" "Current PSI"(w388) -> ()
    n223 = Equal?(x=T1."Fire", y=w360) -> (x = y?=w412:bool)
    n224 = Equal?(x=T1."Arm In", y=w360) -> (x = y?=w406:bool)
    n225 = call "TON.vi"("Delay (ms)"=u32 750 ("Delay ms"), "Input"=w412) -> ("Output"=w410:bool)  [unwired: 9 in]
    n226 = Equal?(x=T1."Clear", y=w360) -> (x = y?=w378:bool)
    n227 = global read "GlobalVariable.vi" "WantToShoot"() -> (w416:bool)
    n228 = global read "GlobalVariable.vi" "Arm State"() -> (w381:bool)
    n229 = global read "GlobalVariable.vi" "ArmOverride"() -> (w397:bool)
    n230 = call "TON.vi"("Delay (ms)"=u32 1500 ("Delay ms"), "Input"=w378) -> ("Output"=w380:bool)  [unwired: 9 in]
    n231 = call "TON.vi"("Delay (ms)"=u32 50 ("Delay ms"), "Input"=w406) -> ("Output"=w404:bool)  [unwired: 9 in]
    n232 = call "TON.vi"("Delay (ms)"=u32 100 ("Delay ms"), "Input"=w397) -> ("Output"=w399:bool)  [unwired: 9 in]
    n233 = call "TON.vi"("Delay (ms)"=u32 1000 ("Delay ms"), "Input"=w381) -> ("Output"=w414:bool)  [unwired: 9 in]
    n234 = call "TON.vi"("Delay (ms)"=u32 250 ("Delay ms"), "Input"=w416) -> ("Output"=w417:bool)  [unwired: 9 in]
    n235 = case shown="\"Arm In\"" w360 {
      selector: w360 -> [w432 w449 w466 w470 w483 w496]
      tunnel: [w433 w450 w457 w474 w475 w506] -> w396
      tunnel: w403 -> [w423 w438 w455 _ _ _]
      tunnel: w417 -> [_ w440 _ _ _ _]
      tunnel: w414 -> [_ _ w462 _ _ _]
      tunnel: w410 -> [_ _ _ w469 _ _]
      tunnel: w408 -> [w427 w441 _ _ w480 _]
      tunnel: w404 -> [_ _ _ _ _ w499]
      tunnel: w399 -> [w426 _ _ _ w479 _]
      tunnel: w400 -> [w422 _ w456 _ _ _]
      tunnel: w380 -> [_ _ _ _ _ _]
      tunnel: [WPI_SolenoidValue."Off" ("Value") WPI_SolenoidValue."Off" ("Value") WPI_SolenoidValue."Off" ("Value") WPI_SolenoidValue."On" ("Value") WPI_SolenoidValue."Off" ("Value") WPI_SolenoidValue."Off" ("Value")] -> w376
      frame "Unready", Default {
        # "Ball PE & Shooter Down & NOT Arm Overide GOTO ARM IN"
        # "Ball PE & Shooter Down & Arm Overide GOTO Ready"
        n236 = Not(x=w426) -> (.not. x?=w424:bool)
        n237 = Compound Arithmetic op=AND(w423, w427, w426) -> (w425:bool)
        n238 = Compound Arithmetic op=AND(w424, w423, w422) -> (w421:bool)
        n239 = Select(t=T1."Arm In", s=w421, f=w432) -> (s? t:f=w431:T1)
        n240 = global write "GlobalVariable.vi" "StateDesiredShooter"(enum16{"None", "Down", "Up"}."None" ("StateDesiredShooter")) -> ()
        n241 = Select(t=T1."Ready", s=w425, f=w431) -> (s? t:f=w433:T1)
        n242 = global write "GlobalVariable.vi" "Underglow"(FALSE ("Underglow")) -> ()
        n243 = global write "GlobalVariable.vi" "ArmInNXTstate"(TRUE ("Poopshtick")) -> ()
        n244 = global write "GlobalVariable.vi" "LogShooting"(FALSE ("Shooting")) -> ()
      }
      frame "Ready" {
        # "If ball sensor is tripped, and Shooter is down,  and button is pushed,\ngo to clear. Starts Shoot Sequence."
        # "If we lose Ball \ngo back to Unready."
        n245 = Compound Arithmetic op=AND(w438, w441, w440) -> (w439:bool)
        n246 = Select(t=T1."Clear", s=w439, f=w449) -> (s? t:f=w445:T1)
        n247 = Select(t=w445, s=w438, f=T1."Unready") -> (s? t:f=w450:T1)
        n248 = global write "GlobalVariable.vi" "StateDesiredShooter"(enum16{"None", "Down", "Up"}."None" ("StateDesiredShooter")) -> ()
        n249 = global write "GlobalVariable.vi" "LogShooting"(FALSE ("Shooting")) -> ()
        n250 = global write "GlobalVariable.vi" "Underglow"(TRUE ("Underglow")) -> ()
      }
      frame "Clear" {
        # "Arm is down and Ball in Shoot Position"
        # "If the ball is lost during the Clear state, the shooter reverts back to\nunready. It's not your fault Drew!"
        n251 = And(x=w456, y=w462) -> (x .and. y?=w461:bool)
        n252 = Not(x=w456) -> (.not. x?=w454:bool)
        n253 = Not(x=w455) -> (.not. x?=w453:bool)
        n254 = And(x=w454, y=w453) -> (x .and. y?=w452:bool)
        n255 = global write "GlobalVariable.vi" "StateDesiredShooter"(enum16{"None", "Down", "Up"}."Down" ("StateDesiredShooter")) -> ()
        n256 = Select(t=T1."Fire", s=w461, f=w466) -> (s? t:f=w458:T1)
        n257 = Select(t=T1."Unready", s=w452, f=w458) -> (s? t:f=w457:T1)
        n258 = global write "GlobalVariable.vi" "LogShooting"(FALSE ("Shooting")) -> ()
        n259 = global write "GlobalVariable.vi" "Underglow"(TRUE ("Underglow")) -> ()
      }
      frame "Fire" {
        # "Wait until done firing to continue."
        n260 = Select(t=T1."Reload", s=w469, f=w470) -> (s? t:f=w474:T1)
        n261 = global write "GlobalVariable.vi" "Underglow"(TRUE ("Underglow")) -> ()
        n262 = global write "GlobalVariable.vi" "LogShooting"(TRUE ("Shooting")) -> ()
        n263 = global write "GlobalVariable.vi" "StateDesiredShooter"(enum16{"None", "Down", "Up"}."None" ("StateDesiredShooter")) -> ()
      }
      frame "Reload" {
        # "Shooter down & Arm Overide GOTO Unready\nShooter down & NOT Arm Overide GOTO ARM IN"
        # "Reload  turns shooter valves off and waits for arm down."
        n264 = Not(x=w479) -> (.not. x?=w486:bool)
        n265 = And(x=w480, y=w486) -> (x .and. y?=w485:bool)
        n266 = And(x=w480, y=w479) -> (x .and. y?=w481:bool)
        n267 = Select(t=T1."Unready", s=w481, f=w483) -> (s? t:f=w482:T1)
        n268 = Select(t=T1."Arm In", s=w485, f=w482) -> (s? t:f=w475:T1)
        n269 = global write "GlobalVariable.vi" "Underglow"(FALSE ("Underglow")) -> ()
        n270 = global write "GlobalVariable.vi" "LogShooting"(FALSE ("Shooting")) -> ()
        n271 = global write "GlobalVariable.vi" "ArmInNXTstate"(FALSE ("Poopshtick")) -> ()
        n272 = global write "GlobalVariable.vi" "StateDesiredShooter"(enum16{"None", "Down", "Up"}."None" ("StateDesiredShooter")) -> ()
      }
      frame "Arm In" {
        # "ARM in Checks Flag ArmInNXTstate if True got to Ready, IF not True go to Unready."
        n273 = global read "GlobalVariable.vi" "ArmInNXTstate"() -> (w493:bool)
        n274 = Equal?(x=w493, y=FALSE) -> (x = y?=w502:bool)
        n275 = Equal?(x=w493, y=TRUE) -> (x = y?=w498:bool)
        n276 = And(x=w502, y=w499) -> (x .and. y?=w501:bool)
        n277 = And(x=w498, y=w499) -> (x .and. y?=w497:bool)
        n278 = global write "GlobalVariable.vi" "LogShooting"(FALSE ("Shooting")) -> ()
        n279 = global write "GlobalVariable.vi" "Underglow"(FALSE ("Underglow")) -> ()
        n280 = global write "GlobalVariable.vi" "StateDesiredShooter"(enum16{"None", "Down", "Up"}."Up" ("StateDesiredShooter")) -> ()
        n281 = Select(t=T1."Ready", s=w497, f=w496) -> (s? t:f=w495:T1)
        n282 = Select(t=T1."Unready", s=w501, f=w495) -> (s? t:f=w506:T1)
      }
    }
    n283 = global write "GlobalVariable.vi" "ShooterCurrentState"(w396) -> ()
    n284 = global read "GlobalVariable.vi" "Fire Override"() -> (w374:bool)
    n285 = Format Into String(format string="%s", w396) -> (resulting string=w393:string)  [unwired: 2 in, 1 out]
    n286 = call <vilib>:"SD Write String.vi"("String"=w393, "Name"="Shooter State") -> ()  [unwired: 8 in, 2 out]
    n287 = global write "GlobalVariable.vi" "ShooterString"(w393) -> ()
    n288 = call "TON.vi"("Delay (ms)"=u32 2000 ("Delay ms"), "Input"=w374) -> ("Output"=w372:bool)  [unwired: 9 in]
    n289 = Select(t=WPI_SolenoidValue."On", s=w372, f=w376) -> (s? t:f=w375:T32)
    n290 = call-poly <vilib>:"WPI_SolenoidSet.vi"("Value"=w375, "SolenoidDevRef"=w377) -> ()  [unwired: 8 in, 2 out]
    n291 = call-poly <vilib>:"WPI_SolenoidSet.vi"("Value"=w375, "SolenoidDevRef"=w370) -> ()  [unwired: 8 in, 2 out]
  }
